vi "LabVIEW2AccData_SWord.vi"(1 "Acc_Data_In":T1[](array[typedef]), 4 "Value":i16) -> (15 "Acc_Data_Out":T1[](array[typedef]))   [LabVIEW 2012, in "ACC_LabVIEW.lvlib"]
uses:
  ACC_LabVIEW.lvlib
  ACC_LabVIEW_Container.ctl
  ACC_LabVIEW_DataTypes.ctl
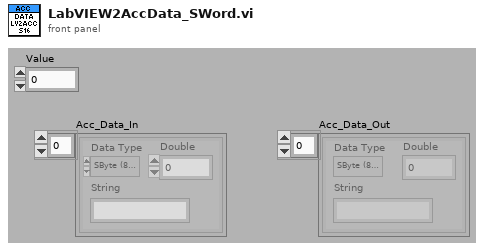
[diagram p1: front panel]
types:
  T1 = typedef "ACC_LabVIEW.lvlib/ACC_LabVIEW_Container.ctl" = cluster{"Data Type":T2, "String":string, "Double":dbl}
  T2 = typedef "ACC_LabVIEW.lvlib/ACC_LabVIEW_DataTypes.ctl" = enum16{"SByte (8Bit Int signed)", "UByte (8Bit int unsigned)", "SWord (16Bit Int signed)", "UWord (16Bit Int unsigned)", "SLong (32Bit Int signed)", "ULong (32Bit Int unsigned)", "Float32 (float)", "Float64 (double)", "String"}
  T3 = cluster{"Data Type":T2, "String":string, "Value":i16}
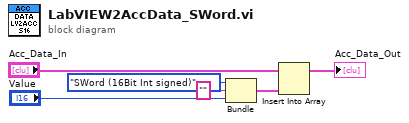
[diagram p0: block diagram]
diagram:
  n1 = Bundle("Data Type"=ACC_LabVIEW_DataTypes."SWord (16Bit Int signed)", "String"="", "Value"="Value") -> (w6:T3)  [unwired: 1 in]
  n2 = Insert Into Array(array="Acc_Data_In", new element=w6) -> (→"Acc_Data_Out":T1[])  [unwired: 1 in]
